vi "soilmo.vi"() -> ()   [LabVIEW 2020]
uses:
  <vilib>/MakerHub/LINX/LMH-LINX.lvlib
  <vilib>/MakerHub/LINX/Public/Peripherals/Analog/Analog Read 1 Chan.vi
  <vilib>/MakerHub/LINX/Public/Peripherals/PWM/PWM Set Duty Cycle 1 Chan.vi
  <vilib>/MakerHub/LINX/Public/Peripherals/Digital/Digital Write 1 Chan.vi
  <vilib>/MakerHub/LINX/Public/Utilities/Open Serial.vi
panel:
  in  "stop for soilmoisture":bool
  out "Waveform Chart moisture":dbl(graph)
  in  "Analog Channe for soil moisturel":u8
  in  "PwmpinLedMoisture":u8
  in  "Pumppin":u8
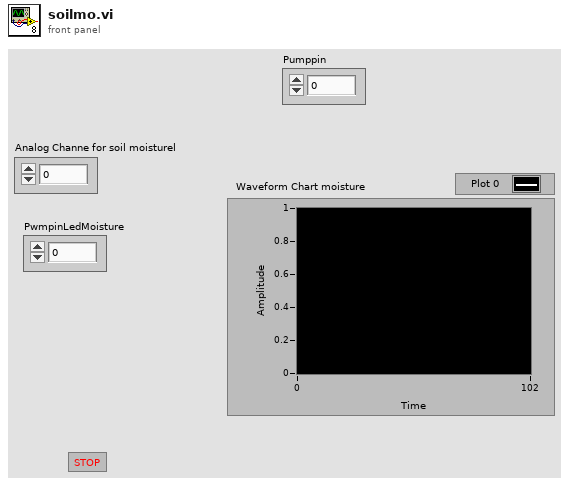
[diagram p1: front panel]
types:
  T1 = typedef "LMH-LINX.lvlib/LINX Ref.ctl" = cluster{"IO":T2, "Interface":T3, "LINX Device Config":T4}
  T2 = typedef "LMH-LINX.lvlib/Platform.ctl" = enum16{"Remote", "Local"}
  T3 = typedef "LMH-LINX.lvlib/Interface.ctl" = enum16{"Serial", "TCP"}
  T4 = typedef "LMH-LINX.lvlib/Device.lvlib/LINX Device Config.ctl" = cluster{"Interface":T3, "COM Port":refnum<visa-resource-name>, "TCP Configuration":T5, "Device Family":u8, "Device ID":u8, "Device Name":string, "TCP Ref":refnum<k5>, "Channels":T6}
  T5 = typedef "LMH-LINX.lvlib/Device.lvlib/TCP Config.ctl" = cluster{"IP Address":string, "Port":u16}
  T6 = typedef "LMH-LINX.lvlib/Channels.ctl" = cluster{"DI":u8[], "DO":u8[], "AI":u8[], "AO":u8[], "PWM":u8[], "QE":u8[], "UART":u8[], "I2C 2":u8[], "SPI":u8[], "CAN":u8[], "Servo":u8[], "AI Ref (V)":dbl, "AI Resolution (Bits)":u8, "AO Ref (V)":dbl, "AO Resolution (Bits)":u8}
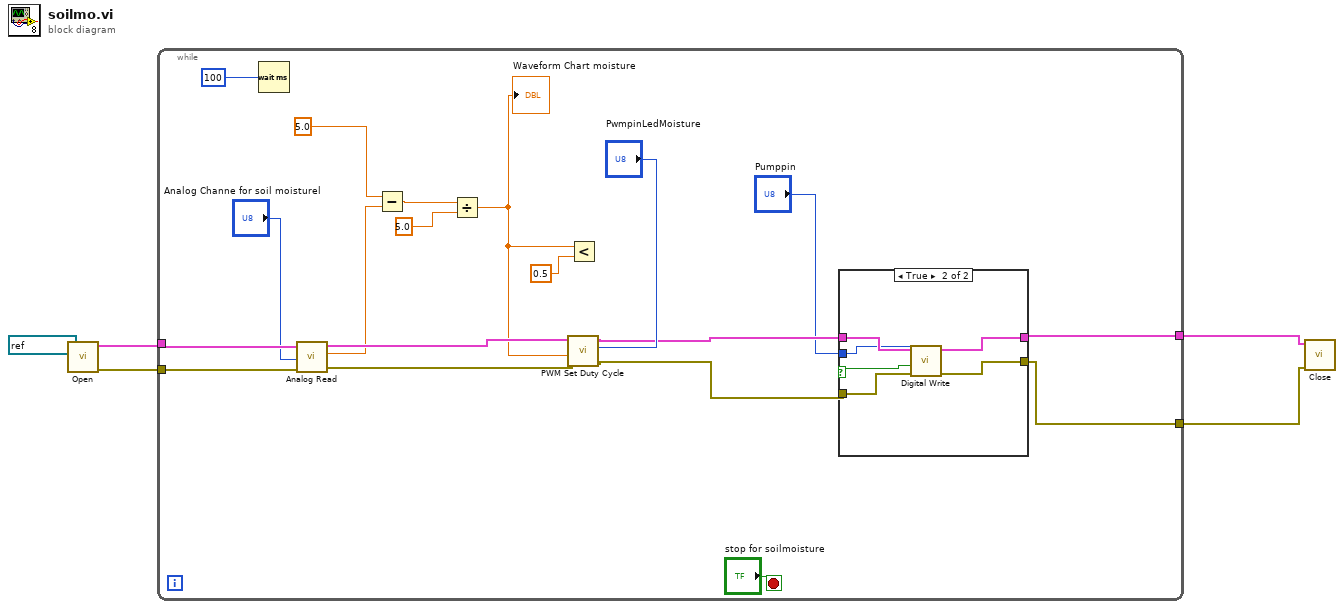
[diagram p0: block diagram]
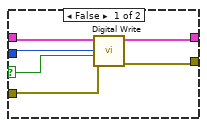
[diagram p2: hidden frame]
diagram:
  n1 = call-poly <vilib>:"Open.vi"("Serial Port"=refnum<visa-resource-name> "COM13") -> ("Error Out"=w4:errorcluster, "LINX Resource"=w5:T1)  [unwired: 8 in, 1 out]
  n2 = while {
    tunnel: [w11] -> w3
    tunnel: w5 -> [w17]
    tunnel: [w10] -> w2
    tunnel: w4 -> [w9]
    stop <- "stop for soilmoisture" stop-if-true
    n3 = Wait (ms)(milliseconds to wait=u32 100 ("millisecond timer value")) -> ()  [unwired: 1 out]
    n4 = call-poly <vilib>:"Analog Read.vi"("Error In"=w9, "Analog Channel"="Analog Channe for soil moisturel", "LINX Resource"=w17) -> ("Error Out"=w22:errorcluster, "Voltage"=w21:dbl, "LINX Resource"=w23:T1)  [unwired: 5 in, 1 out]
    n5 = Subtract(x=5.0, y=w21) -> (x-y=w19:dbl)
    n6 = Divide(x=w19, y=5.0) -> (x/y=w8:dbl)
    "Waveform Chart moisture" <- w8
    n7 = call-poly <vilib>:"PWM Set Duty Cycle.vi"("Error In"=w22, "Duty Cycle (0-1)"=w8, "PWM Channel"="PwmpinLedMoisture", "LINX Resource"=w23) -> ("Error Out"=w13:errorcluster, "LINX Resource"=w14:T1)  [unwired: 6 in]
    n8 = Less?(x=w8, y=0.5) -> ()  [unwired: 1 out]
    n9 = case shown="True" w6 {
      selector: [w27 w33] -> w6
      tunnel: w14 -> [w31 w37]
      tunnel: [w30 w36] -> w11
      tunnel: w13 -> [w28 w35]
      tunnel: [w29 w34] -> w10
      tunnel: "Pumppin" -> [w26 w32]
      frame False {
        n10 = call-poly <vilib>:"Digital Write.vi"("Error In"=w28, "Output Value"=w27, "DO Channel"=w26, "LINX Resource"=w31) -> ("Error Out"=w29:errorcluster, "LINX Resource"=w30:T1)  [unwired: 6 in]
      }
      frame True {
        n11 = call-poly <vilib>:"Digital Write.vi"("Error In"=w35, "Output Value"=w33, "DO Channel"=w32, "LINX Resource"=w37) -> ("Error Out"=w34:errorcluster, "LINX Resource"=w36:T1)  [unwired: 6 in]
      }
    }
  }
  n12 = call <vilib>:"Close.vi"("Error In"=w2, "LINX Resource"=w3) -> ()  [unwired: 9 in, 1 out]
